vi "Simple While Loop Counter (LV 2013).vi"(9 "Stop":bool, 10 "Reset":bool, 11 "Count Direction":enum16{"Count Down", "Count Up"}(ring)=enum."Count Up") -> (3 "Count":u32)   [LabVIEW 2023]
doc: "This VI is an example of how you can implement a counter using a while loop. The count value will either increase or decreases (based on selected enum control) its value each loop iteration. The count value will continue to increase or decreases unless the user resets the count, changes count direction, or stops the VI."
panel:
  # "This VI is an example of how you can implement a counter using a while loop. The count value will either increase or decreases (based on selected enum control) its value each loop iteration. The count value will continue to increase or decreases unless the user resets the count, changes count direction, or stops the VI."
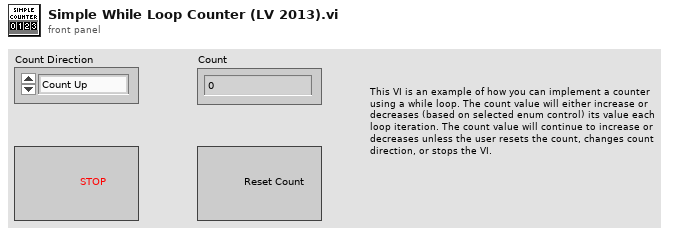
[diagram p1: front panel]
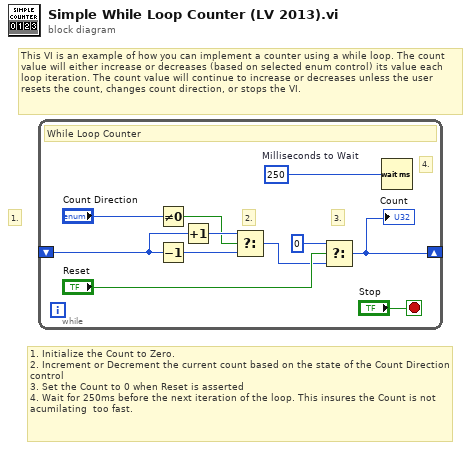
[diagram p0: block diagram]
diagram:
  # "This VI is an example of how you can implement a counter using a while loop. The count value will either increase or decreases (based on selected enum control) its value each loop iteration. The count value will continue to increase or decreases unless the user resets the count, changes count direction, or stops the VI."
  # "1."
  # "1. Initialize the Count to Zero.\n2. Increment or Decrement the current count based on the state of the Count Direction control\n3. Set the Count to 0 when Reset is asserted \n4. Wait for 250ms before the next iteration of the loop. This insures the Count is not acumilating  too fast."
  n1 = while "Timed Loop" {
    shift-right: [w11] -> _
    shift-left: _ -> [w6]
    stop <- "Stop" stop-if-true
    w1 = u32 250  # Milliseconds to Wait
    # "4."
    # "3."
    # "2."
    # "While Loop Counter"
    n2 = Not Equal To 0?(x="Count Direction") -> (x != 0?=w3:bool)
    n3 = Decrement(x=w6) -> (x-1=w7:u32)
    n4 = Increment(x=w6) -> (x+1=w5:u32)
    n5 = Select(t=w5, s=w3, f=w7) -> (s? t:f=w2:u32)
    n6 = Select(t=u32 0, s="Reset", f=w2) -> (s? t:f=w11:u32)
    "Count" <- w11
    n7 = Wait (ms)(milliseconds to wait=w1) -> ()  [unwired: 1 out]
  }
